vi "ToolModGLOB.vi"() -> ()   [LabVIEW 2015, in "Tool Module.lvlib"]
uses:
  Tool Module.lvlib
  Tool Typedefs/_Data Stream Fmt Params Cluster--typedef.ctl
  Tool Typedefs/_FPGA Setup Params Cluster--typedef.ctl
  Tool Typedefs/_FPGA Timing Constraints Cluster--typedef.ctl
  Tool Typedefs/_FPGA Timing Ctrl Cluster--typedef.ctl
  Tool Typedefs/_FPGA Laser Config Cluster--typedef.ctl
  Tool Typedefs/_FPGA Peak Proc Cfg Cluster--typedef.ctl
  Tool Typedefs/_FPGA SPI Cfg Cluster--typedef.ctl
panel:
  in  "Mtr Ctrl Reg(File)":u16=350 format="%09b"
  in  "Mtr Ctrl Reg(temp)":u16=350 format="%09b"
  in  "Version String":string
  in  "FPGA Setup Parameters":T1={"FPGA Timing Constraints"={"frame.length Min"=530, "frame.ST_OFF Min"=15, "frame.ST_ON Min"=8, "frame.first data idx"=14, "frame.integ Offset"=6, "frame.integ Delay"=3, "frame.ad_latch Delay"=11, "frame.trig time Max"=0}, "FPGA Timing Ctrl"={"trig.time"=220, "integ.count 1"=400, "integ.count 2"=350, "encdr.latch ctrl"=1, "pixel.read count"=512, "clock.select"=2, "ad.clock offset"=16, "data.control reg"=2}, "FPGA Laser Config"={"laser.gain"=10, "laser.threshold Low"=1400, "laser.threshold High"=1900, "laser.dac init"=912, "laser.dac Min"=800, "laser.dac Max"=4000, "laser.config reg"=3}, "FPGA Peak Proc Cfg"={"PD.threshold"=0, "PD.width detect Min"=0, "PD.sensor pixels"=512, "PD.config reg"=23}, "FPGA SPI Cfg"={"SPI Divide Value"=1, "SPI config reg"=1}} {"FPGA SPI Cfg"."SPI config reg" format="%03b"; "FPGA Peak Proc Cfg"."PD.config reg" format="%05b"; "FPGA Laser Config"."laser.config reg" format="%02b"; "FPGA Timing Ctrl"."data.control reg" format="%03b"; "FPGA Timing Constraints"."frame.trig time Max" format="%0.0f"}
  in  "Tool Config Filename":string="QC-X Tool Config.xml"
  in  "Inspect Range Cnt Max":i32=50
  in  "Wait Motion Count Max":i32=50
  in  "Homing Loop MotionTimeout (sec)":i32=5
  out "Connected?":bool
  in  "Data Stream Fmt Params":T7={"Samples per Block"=20, "Raw Data Status Len"=0, "Fltr Data Status Len"=0}
  out "Cfg Data from Tool OK?":bool
  out "Tool Cfg File OK?":bool
  in  "In Range Tolerance":i32=40000
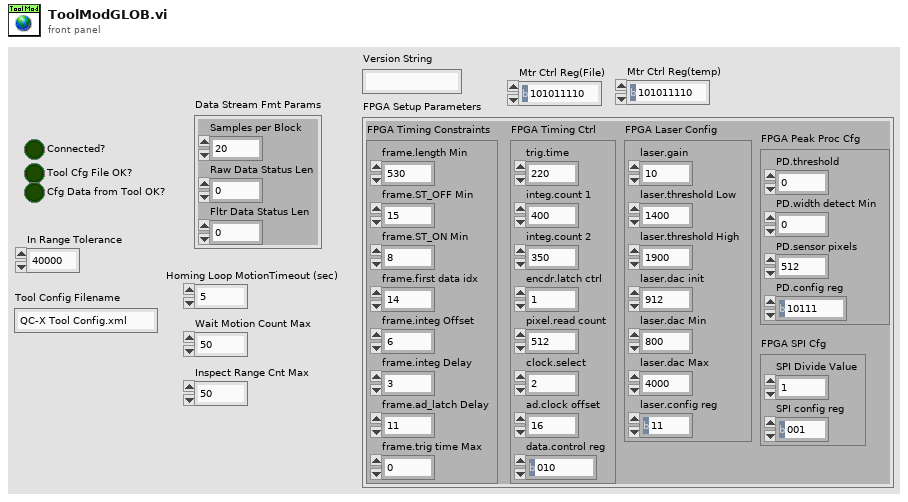
[diagram p1: front panel]
types:
  T1 = typedef "_FPGA Setup Params Cluster--typedef.ctl" = cluster{"FPGA Timing Constraints":T2, "FPGA Timing Ctrl":T3, "FPGA Laser Config":T4, "FPGA Peak Proc Cfg":T5, "FPGA SPI Cfg":T6}
  T2 = typedef "_FPGA Timing Constraints Cluster--typedef.ctl" = cluster{"frame.length Min":u16, "frame.ST_OFF Min":u16, "frame.ST_ON Min":u16, "frame.first data idx":u16, "frame.integ Offset":u16, "frame.integ Delay":u16, "frame.ad_latch Delay":u16, "frame.trig time Max":u32}
  T3 = typedef "_FPGA Timing Ctrl Cluster--typedef.ctl" = cluster{"trig.time":u32, "integ.count 1":u32, "integ.count 2":u32, "encdr.latch ctrl":u32, "pixel.read count":u16, "clock.select":u16, "ad.clock offset":u16, "data.control reg":u16}
  T4 = typedef "_FPGA Laser Config Cluster--typedef.ctl" = cluster{"laser.gain":i16, "laser.threshold Low":u16, "laser.threshold High":u16, "laser.dac init":u16, "laser.dac Min":u16, "laser.dac Max":u16, "laser.config reg":u16}
  T5 = typedef "_FPGA Peak Proc Cfg Cluster--typedef.ctl" = cluster{"PD.threshold":u16, "PD.width detect Min":u8, "PD.sensor pixels":u16, "PD.config reg":u16}
  T6 = typedef "_FPGA SPI Cfg Cluster--typedef.ctl" = cluster{"SPI Divide Value":u8, "SPI config reg":u16}
  T7 = typedef "_Data Stream Fmt Params Cluster--typedef.ctl" = cluster{"Samples per Block":i32, "Raw Data Status Len":i32, "Fltr Data Status Len":i32}
diagram:
